vi "Example LabVIEW Table.vi"() -> ()   [LabVIEW 2014]
uses:
  DataGridView/DataGridView.lvclass
panel:
  in  "# of Rows":i32=15
  out "Table Control":string[][](table)
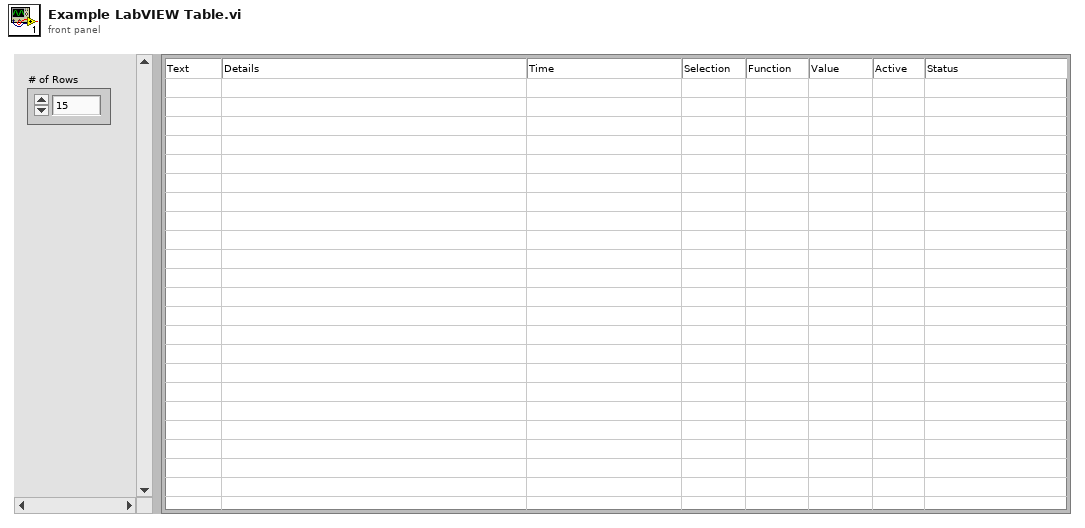
[diagram p1: front panel]
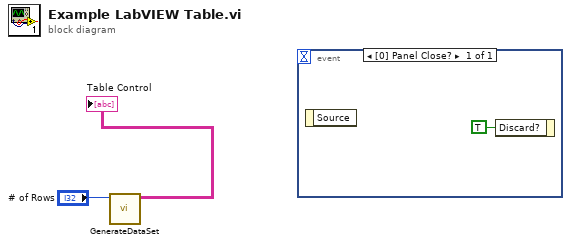
[diagram p0: block diagram]
diagram:
  n1 = call "GenerateDataSet.vi"("Records"="# of Rows") -> ("DataGrid"=→"Table Control":string[][])  [unwired: 10 in]
  n2 = event shown="[0] Panel Close?" {
    selector: _ -> [_]
    dyn-events: _ -> [_]
    timeout: _ -> [_]
    event Panel Close? {
      n3 = event-data() -> ()  [unwired: 1 in, 1 out]
      n4 = event-data("Discard?"=TRUE) -> ()  [unwired: 1 in, 1 out]
    }
  }
